vi "1_Blink_Direct.vi"() -> ()   [LabVIEW 2012]
panel:
  out "BotSpeak":string="SET DIO[0],1\nSET DIO[0],0\nSET DIO[0],1\nSET DIO[0],0\n\n"
  out "expected response":string="1\r\n0\r\n1\r\n0\r\n"
  out "response":string="1\r\n0\r\n1\r\n0\r\n"
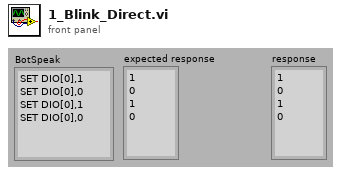
[diagram p1: front panel]
types:
  T1 = typedef "BotSpeak_Control.ctl" = cluster{"Address":string, "Reply EOF":string, "Hardware":path, "Retries":i8, "Timeout":i32}
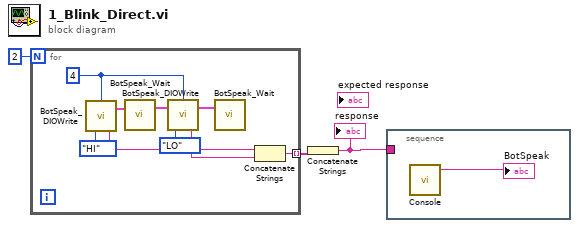
[diagram p0: block diagram]
diagram:
  n1 = for {
    N: 2 -> [_]
    tunnel: [w4] -> w2 mode=indexing
    w9 = u32 4 ("DIO Line")
    n2 = call <userlib>:"BotSpeak_DIOWrite.vi"("State"=enum32{"LO", "HI"}."HI", "DIO Line"=w9) -> ("response"=w6:string, "Bot Settings"=w12:T1)  [unwired: 1 in]
    n3 = call <userlib>:"BotSpeak_Wait.vi"("Bot Settings"=w12) -> ("Bot Settings"=w11:T1)  [unwired: 2 in]
    n4 = call <userlib>:"BotSpeak_DIOWrite.vi"("State"=enum32{"LO", "HI"}."LO", "Bot Settings"=w11, "DIO Line"=w9) -> ("response"=w5:string, "Bot Settings"=w10:T1)
    n5 = call <userlib>:"BotSpeak_Wait.vi"("Bot Settings"=w10) -> ()  [unwired: 2 in, 1 out]
    n6 = Concatenate Strings(w6, w5) -> (w4:string)
  }
  n7 = Concatenate Strings(w2) -> (w1:string)
  "response" <- w1
  n8 = stacked-sequence {
    tunnel: w1 -> [_]
    frame #0 {
      n9 = call <userlib>:"Console.vi"() -> ("BotSpeak"=→"BotSpeak":string)  [unwired: 4 in, 1 out]
    }
  }
